vi "Load LVS EMA 2010b.vi"(10 "Data OUT in":T1={"Impulse Positions"=[], "Old Impulse positions for Undo"=[], "No. Imp"=0, "Parameter Time Series"=[], "Parameter Impuls Series"=[], "Experiment Parameters"={"Freq"=0.0, "Vel"=0, "Acc"=0, "Stimulus"=""}, "Autosort File"=refnum, "Data File"={"Data Channels"=[], "Sample Rate"=0, "Channel List"=[]}, "Experiment data path"=path "", "Image data path"=path "", "LVS data path"=path "", "Raw copy path"=path "", "filename"="", "desaccading parameters"={"Tolerance"=0, "Acc Range"=0.0, "Sample Rate"=0, "Impulse Plane 2"=enum."Other", "Impulse dir"=FALSE}, "Experiment Parameters 2"={"Subject"="", "Strain"="", "Rotation plane"="", "Experimenter"="", "Trial"=0.0, "Time"=0.0}, "Excel"={"Excel._Application"=refnum, "Use Excel"=FALSE, "Worksheet SINE"=refnum, "Row SINE"=0, "Worksheet TRANS"=refnum, "Row TRANS"=0}, "Session Config File"=refnum, "Autosort Parameter Set"=0, "EMA Version"="", "desacc "={"Threshold 1 [Acc]"=0.0, "Threshold 2 [% of TH1]"=0, "tolerance"=0, "Search WD "=0.0, " always use TH2"=FALSE, "Range"=0.0, "Max time"=0.0, "Min time"=0.0, "Velocity Threshold"=0}, "Cycle Nr for Saccades"={"POS"=0, "NEG"=0}, "Undo Counter"=0, "History Length"=0, "Redo Counter"=0, "Histpry Position"=0, "Raw Data File"={"Data Channels"=[], "Sample Rate"=0, "Channel List"=[]}, "calibration name"="No file selected"} {"Parameter Time Series"."time offset" format="%.3f"; "Parameter Time Series"."Gain" format="%.1f"; "Parameter Time Series"."Offset" format="%.1f"; "Parameter Time Series"."List 1" items=["Motor-Pos", "Motor-Vel", "Lx Position-in-Head", "Ly Position-in-Head", "Lz Position-in-Head", "Lx Velocity-in-Head", "Ly Velocity-in-Head", "Lz Velocity-in-Head", "Ll Velocity-in-Head", "Lr Velocity-in-Head", "Lx Accel-in-Head", "Ly Accel-in-Head", "Lz Accel-in-Head", "Rx Position-in-Head", "Ry Position-in-Head", "Rz Position-in-Head", "Rx Velocity-in-Head", "Ry Velocity-in-Head", "Rz Velocity-in-Head", "Rl Velocity-in-Head", "Rr Velocity-in-Head", "Rx Accel-in-Head", "Ry Accel-in-Head", "Rz Accel-in-Head", "Global Trigger", "", "", ""]; "Parameter Impuls Series"."Gain" format="%.1f"; "Parameter Impuls Series"."Offset" format="%.1f"}, 11 "Byte Stream File in":refnum<file>) -> (2 "Byte Stream File out":refnum<file>, 3 "Data OUT out":T1={"Impulse Positions"=[], "Old Impulse positions for Undo"=[], "No. Imp"=0, "Parameter Time Series"=[], "Parameter Impuls Series"=[], "Experiment Parameters"={"Freq"=0.0, "Vel"=0, "Acc"=0, "Stimulus"=""}, "Autosort File"=refnum, "Data File"={"Data Channels"=[], "Sample Rate"=0, "Channel List"=[]}, "Experiment data path"=path "", "Image data path"=path "", "LVS data path"=path "", "Raw copy path"=path "", "filename"="", "desaccading parameters"={"Tolerance"=0, "Acc Range"=0.0, "Sample Rate"=0, "Impulse Plane 2"=enum."Other", "Impulse dir"=FALSE}, "Experiment Parameters 2"={"Subject"="", "Strain"="", "Rotation plane"="", "Experimenter"="", "Trial"=0.0, "Time"=0.0}, "Excel"={"Excel._Application"=refnum, "Use Excel"=FALSE, "Worksheet SINE"=refnum, "Row SINE"=0, "Worksheet TRANS"=refnum, "Row TRANS"=0}, "Session Config File"=refnum, "Autosort Parameter Set"=0, "EMA Version"="", "desacc "={"Threshold 1 [Acc]"=0.0, "Threshold 2 [% of TH1]"=0, "tolerance"=0, "Search WD "=0.0, " always use TH2"=FALSE, "Range"=0.0, "Max time"=0.0, "Min time"=0.0, "Velocity Threshold"=0}, "Cycle Nr for Saccades"={"POS"=0, "NEG"=0}, "Undo Counter"=0, "History Length"=0, "Redo Counter"=0, "Histpry Position"=0, "Raw Data File"={"Data Channels"=[], "Sample Rate"=0, "Channel List"=[]}, "calibration name"="No file selected"} {"Parameter Time Series"."time offset" format="%.3f"; "Parameter Time Series"."Gain" format="%.1f"; "Parameter Time Series"."Offset" format="%.1f"; "Parameter Time Series"."List 1" items=["Motor-Pos", "Motor-Vel", "Lx Position-in-Head", "Ly Position-in-Head", "Lz Position-in-Head", "Lx Velocity-in-Head", "Ly Velocity-in-Head", "Lz Velocity-in-Head", "Ll Velocity-in-Head", "Lr Velocity-in-Head", "Lx Accel-in-Head", "Ly Accel-in-Head", "Lz Accel-in-Head", "Rx Position-in-Head", "Ry Position-in-Head", "Rz Position-in-Head", "Rx Velocity-in-Head", "Ry Velocity-in-Head", "Rz Velocity-in-Head", "Rl Velocity-in-Head", "Rr Velocity-in-Head", "Rx Accel-in-Head", "Ry Accel-in-Head", "Rz Accel-in-Head", "Global Trigger", "", "", ""]; "Parameter Impuls Series"."Gain" format="%.1f"; "Parameter Impuls Series"."Offset" format="%.1f"})   [LabVIEW 2014]
uses:
  type-defs/TD_Statemachine-Data.ctl
  type-defs/TD_Time Series.ctl
  type-defs/TD_Impulse Parameter.ctl
  core.lvlib
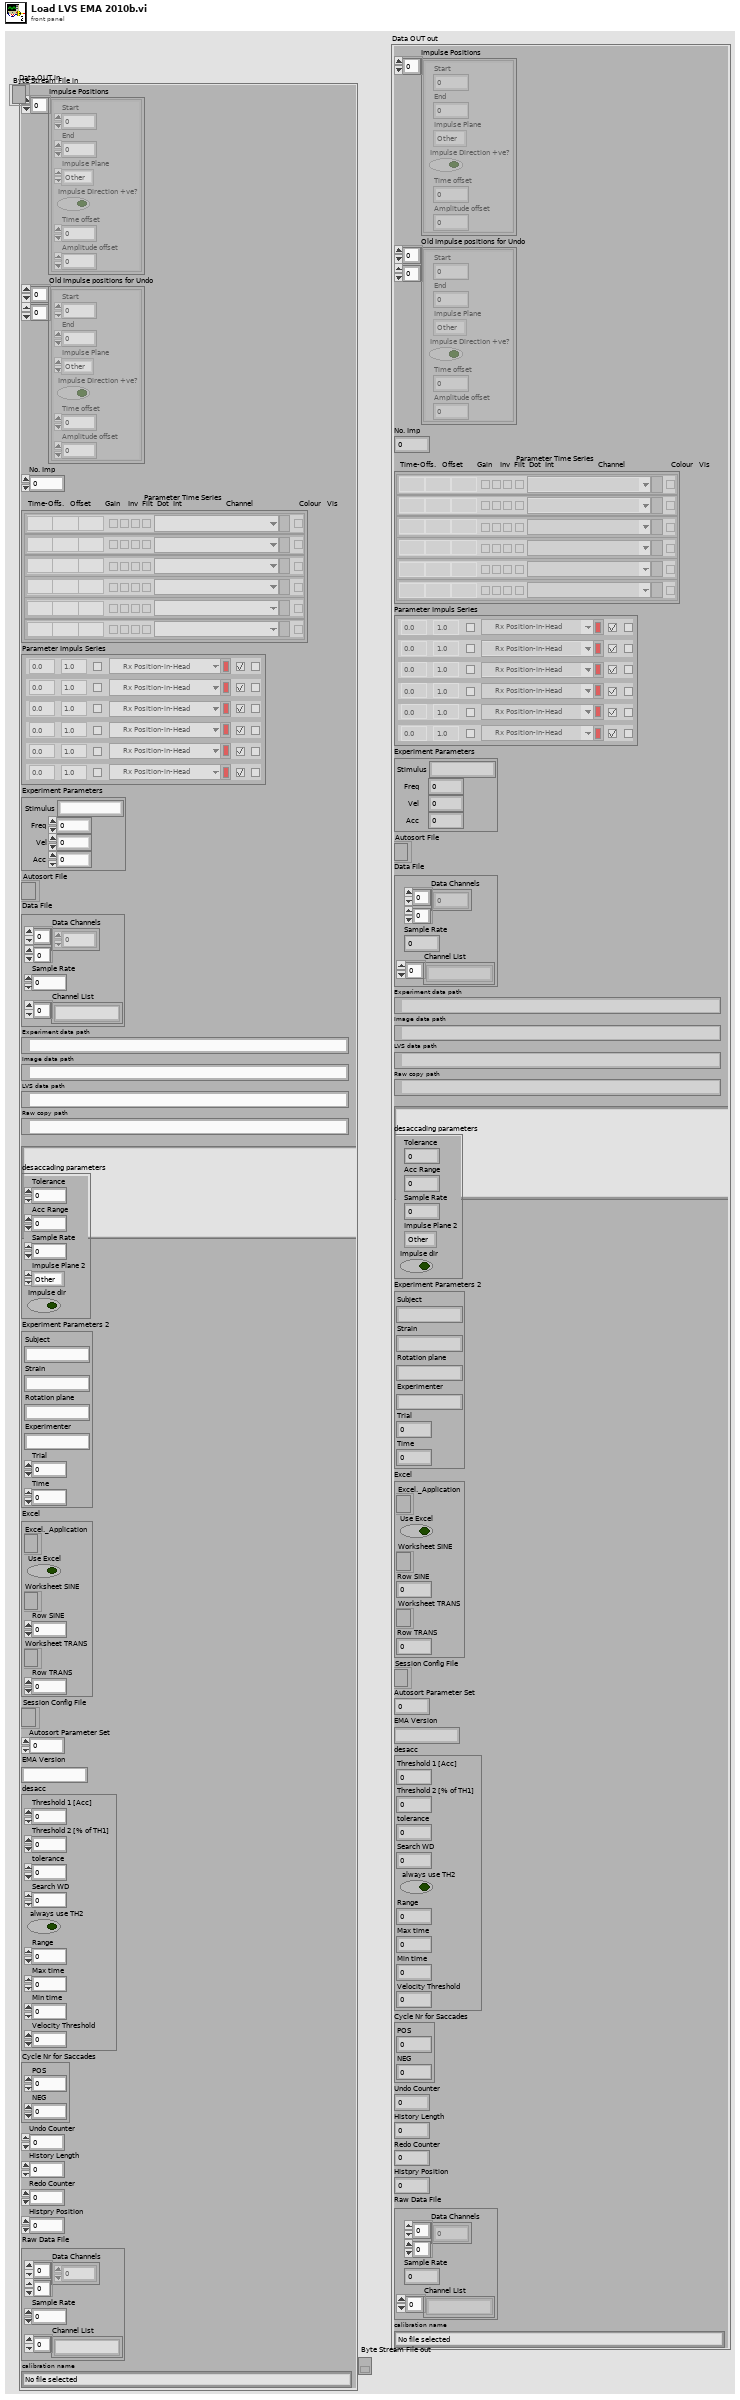
[diagram p1: front panel]
types:
  T1 = typedef "core.lvlib/TD_Statemachine-Data.ctl" = cluster{"Impulse Positions":cluster{"Start":i32, "End":i32, "Impulse Plane":enum16{"Other", "Yaw", "Pitch", "Roll", "LARP", "RALP"}, "Impulse Direction +ve?":bool, "Time offset":i32, "Amplitude offset":dbl}[], "Old Impulse positions for Undo":cluster{"Start":i32, "End":i32, "Impulse Plane":enum16{"Other", "Yaw", "Pitch", "Roll", "LARP", "RALP"}, "Impulse Direction +ve?":bool, "Time offset":i32, "Amplitude offset":dbl}[][], "No. Imp":i32, "Parameter Time Series":T2, "Parameter Impuls Series":T3, "Experiment Parameters":cluster{"Freq":dbl, "Vel":i32, "Acc":i32, "Stimulus":string}, "Autosort File":refnum<file>, "Data File":cluster{"Data Channels":dbl[][], "Sample Rate":i32, "Channel List":string[]}, "Experiment data path":path, "Image data path":path, "LVS data path":path, "Raw copy path":path, "filename":string, "desaccading parameters":cluster{"Tolerance":i32, "Acc Range":dbl, "Sample Rate":i32, "Impulse Plane 2":enum16{"Other", "Yaw", "Pitch", "Roll", "LARP", "RALP"}, "Impulse dir":bool}, "Experiment Parameters 2":cluster{"Subject":string, "Strain":string, "Rotation plane":string, "Experimenter":string, "Trial":dbl, "Time":dbl}, "Excel":cluster{"Excel._Application":refnum<k7>, "Use Excel":bool, "Worksheet SINE":refnum<k7>, "Row SINE":i32, "Worksheet TRANS":refnum<k7>, "Row TRANS":i32}, "Session Config File":refnum<file>, "Autosort Parameter Set":i32, "EMA Version":string, "desacc ":cluster{"Threshold 1 [Acc]":dbl, "Threshold 2 [% of TH1]":i32, "tolerance":i32, "Search WD ":dbl, " always use TH2":bool, "Range":dbl, "Max time":dbl, "Min time":dbl, "Velocity Threshold":i32}, "Cycle Nr for Saccades":cluster{"POS":i32, "NEG":i32}, "Undo Counter":i32, "History Length":i32, "Redo Counter":i32, "Histpry Position":i32, "Raw Data File":cluster{"Data Channels":dbl[][], "Sample Rate":i32, "Channel List":string[]}, "calibration name":string}
  T2 = typedef "core.lvlib/TD_Time Series.ctl" = cluster{"time offset":dbl, "Offset":dbl, "Gain":dbl, "inverse":bool, "filter data":bool, "dots":bool, "interpolate":bool, "List 1":u16, "Color Box":u32, "Boolean":bool}[]
  T3 = typedef "core.lvlib/TD_Impulse Parameter.ctl" = cluster{"Color":u32, "Visible":bool, "Channel":u16, "Invert":bool, "Desaccade":bool, "Offset":dbl, "Gain":dbl}[]
  T4 = cluster{"Data Channels":dbl[][], "Sample Rate":i32, "Channel List":string[]}
  T5 = cluster{"Data Output":cluster{"Data Channels":dbl[][], "Sample Rate":i32, "Channel List":string[]}, "Data OUT in":T1}
  T6 = cluster{"Start":i32, "End":i32, "Impulse Plane":enum16{"Other", "Yaw", "Pitch", "Roll", "LARP", "RALP"}, "Impulse Direction +ve?":bool, "Time offset":i32, "Amplitude offset":dbl}[]
  T7 = cluster{"Start":i32, "End":i32, "Impulse Plane":enum16{"Other", "Yaw", "Pitch", "Roll", "LARP", "RALP"}, "Impulse Direction +ve?":bool, "Time offset":i32, "Amplitude offset":dbl}[][]
  T8 = cluster{"Freq":dbl, "Vel":i32, "Acc":i32, "Stimulus":string}
  T9 = cluster{"Tolerance":i32, "Acc Range":dbl, "Sample Rate":i32, "Impulse Plane 2":enum16{"Other", "Yaw", "Pitch", "Roll", "LARP", "RALP"}, "Impulse dir":bool}
  T10 = cluster{"Subject":string, "Strain":string, "Rotation plane":string, "Experimenter":string, "Trial":dbl, "Time":dbl}
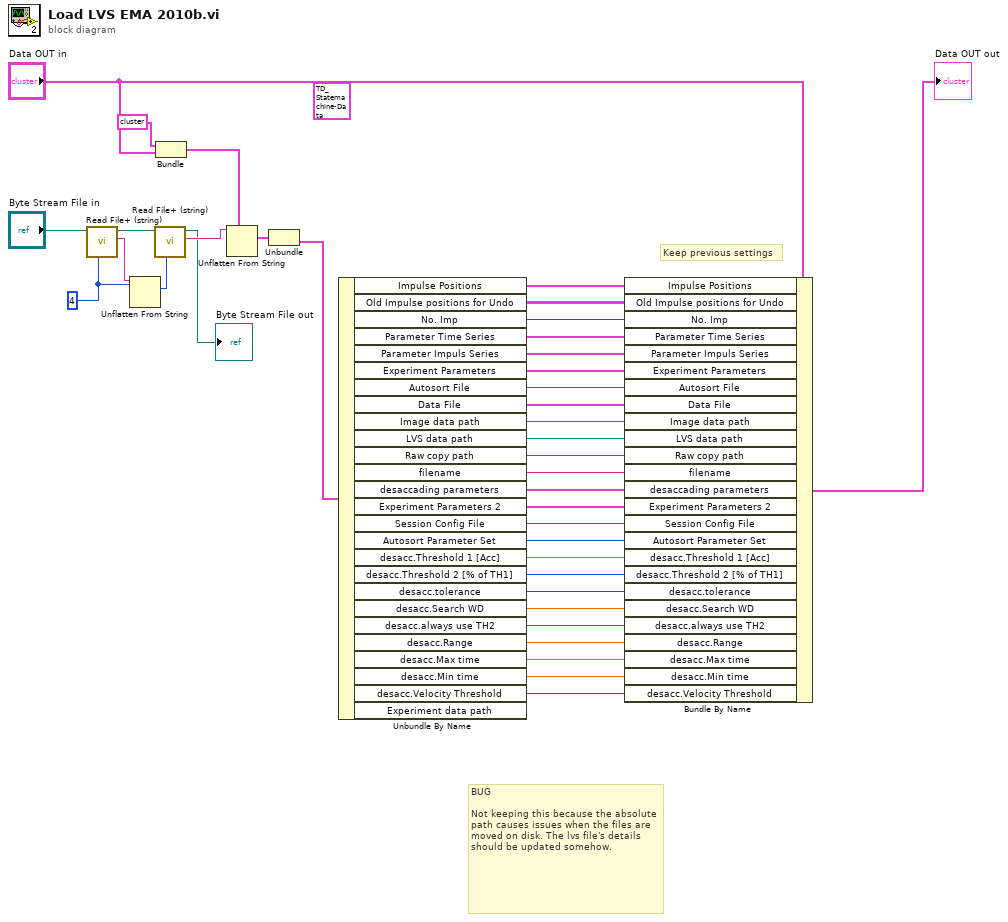
[diagram p0: block diagram]
diagram:
  (unwired) T1 {"Impulse Positions"=[{"Start"=4942, "End"=5034, "Impulse Plane"=enum."Yaw", "Impulse Direction +ve?"=TRUE, "Time offset"=0, "Amplitude offset"=0.0}, {"Start"=5524, "End"=5615, "Impulse Plane"=enum."Yaw", "Impulse Direction +ve?"=FALSE, "Time offset"=0, "Amplitude offset"=0.0}, {"Start"=6320, "End"=6414, "Impulse Plane"=enum."Yaw", "Impulse Direction +ve?"=FALSE, "Time offset"=0, "Amplitude offset"=0.0}, {"Start"=6789, "End"=6880, "Impulse Plane"=enum."Yaw", "Impulse Direction +ve?"=TRUE, "Time offset"=0, "Amplitude offset"=0.0}, {"Start"=7275, "End"=7365, "Impulse Plane"=enum."Yaw", "Impulse Direction +ve?"=FALSE, "Time offset"=0, "Amplitude offset"=0.0}, {"Start"=7765, "End"=7854, "Impulse Plane"=enum."Yaw", "Impulse Direction +ve?"=FALSE, "Time offset"=0, "Amplitude offset"=0.0}, {"Start"=8262, "End"=8354, "Impulse Plane"=enum."Yaw", "Impulse Direction +ve?"=TRUE, "Time offset"=0, "Amplitude offset"=0.0}, {"Start"=9102, "End"=9192, "Impulse Plane"=enum."Yaw", "Impulse Direction +ve?"=TRUE, "Time offset"=0, "Amplitude offset"=0.0}, {"Start"=9641, "End"=9736, "Impulse Plane"=enum."Yaw", "Impulse Direction +ve?"=FALSE, "Time offset"=0, "Amplitude offset"=0.0}, {"Start"=10150, "End"=10242, "Impulse Plane"=enum."Yaw", "Impulse Direction +ve?"=FALSE, "Time offset"=0, "Amplitude offset"=0.0}, {"Start"=10613, "End"=10703, "Impulse Plane"=enum."Yaw", "Impulse Direction +ve?"=TRUE, "Time offset"=0, "Amplitude offset"=0.0}, {"Start"=11147, "End"=11237, "Impulse Plane"=enum."Yaw", "Impulse Direction +ve?"=TRUE, "Time offset"=0, "Amplitude offset"=0.0}, {"Start"=11689, "End"=11781, "Impulse Plane"=enum."Yaw", "Impulse Direction +ve?"=TRUE, "Time offset"=0, "Amplitude offset"=0.0}, {"Start"=12321, "End"=12416, "Impulse Plane"=enum."Yaw", "Impulse Direction +ve?"=FALSE, "Time offset"=0, "Amplitude offset"=0.0}, {"Start"=12810, "End"=12901, "Impulse Plane"=enum."Yaw", "Impulse Direction +ve?"=FALSE, "Time offset"=0, "Amplitude offset"=0.0}, {"Start"=13306, "End"=13397, "Impulse Plane"=enum."Yaw", "Impulse Direction +ve?"=FALSE, "Time offset"=0, "Amplitude offset"=0.0}, {"Start"=13888, "End"=13980, "Impulse Plane"=enum."Yaw", "Impulse Direction +ve?"=TRUE, "Time offset"=0, "Amplitude offset"=0.0}, {"Start"=14402, "End"=14493, "Impulse Plane"=enum."Yaw", "Impulse Direction +ve?"=FALSE, "Time offset"=0, "Amplitude offset"=0.0}, {"Start"=14971, "End"=15063, "Impulse Plane"=enum."Yaw", "Impulse Direction +ve?"=FALSE, "Time offset"=0, "Amplitude offset"=0.0}, {"Start"=15459, "End"=15553, "Impulse Plane"=enum."Yaw", "Impulse Direction +ve?"=TRUE, "Time offset"=0, "Amplitude offset"=0.0}, {"Start"=16020, "End"=16112, "Impulse Plane"=enum."Yaw", "Impulse Direction +ve?"=FALSE, "Time offset"=0, "Amplitude offset"=0.0}, {"Start"=16530, "End"=16622, "Impulse Plane"=enum."Yaw", "Impulse Direction +ve?"=TRUE, "Time offset"=0, "Amplitude offset"=0.0}, {"Start"=17204, "End"=17295, "Impulse Plane"=enum."Yaw", "Impulse Direction +ve?"=TRUE, "Time offset"=0, "Amplitude offset"=0.0}, {"Start"=17830, "End"=17921, "Impulse Plane"=enum."Yaw", "Impulse Direction +ve?"=FALSE, "Time offset"=0, "Amplitude offset"=0.0}, {"Start"=19274, "End"=19361, "Impulse Plane"=enum."Yaw", "Impulse Direction +ve?"=FALSE, "Time offset"=0, "Amplitude offset"=0.0}, {"Start"=19884, "End"=19973, "Impulse Plane"=enum."Yaw", "Impulse Direction +ve?"=FALSE, "Time offset"=0, "Amplitude offset"=0.0}, {"Start"=20423, "End"=20518, "Impulse Plane"=enum."Yaw", "Impulse Direction +ve?"=TRUE, "Time offset"=0, "Amplitude offset"=0.0}, {"Start"=21003, "End"=21091, "Impulse Plane"=enum."Yaw", "Impulse Direction +ve?"=FALSE, "Time offset"=0, "Amplitude offset"=0.0}, {"Start"=21526, "End"=21619, "Impulse Plane"=enum."Yaw", "Impulse Direction +ve?"=FALSE, "Time offset"=0, "Amplitude offset"=0.0}, {"Start"=22032, "End"=22124, "Impulse Plane"=enum."Yaw", "Impulse Direction +ve?"=TRUE, "Time offset"=0, "Amplitude offset"=0.0}, {"Start"=22661, "End"=22752, "Impulse Plane"=enum."Yaw", "Impulse Direction +ve?"=FALSE, "Time offset"=0, "Amplitude offset"=0.0}, {"Start"=23810, "End"=23900, "Impulse Plane"=enum."Yaw", "Impulse Direction +ve?"=TRUE, "Time offset"=0, "Amplitude offset"=0.0}], "Old Impulse positions for Undo"=[], "No. Imp"=18, "Parameter Time Series"=[{"time offset"=0.0, "Offset"=0.0, "Gain"=1.0, "inverse"=FALSE, "filter data"=FALSE, "dots"=FALSE, "interpolate"=FALSE, "List 1"=1, "Color Box"=65295, "Boolean"=TRUE}, {"time offset"=0.0, "Offset"=0.0, "Gain"=1.0, "inverse"=FALSE, "filter data"=FALSE, "dots"=FALSE, "interpolate"=FALSE, "List 1"=13, "Color Box"=16777224, "Boolean"=TRUE}, {"time offset"=0.0, "Offset"=0.0, "Gain"=1.0, "inverse"=FALSE, "filter data"=FALSE, "dots"=FALSE, "interpolate"=FALSE, "List 1"=6, "Color Box"=6618880, "Boolean"=FALSE}, {"time offset"=0.0, "Offset"=0.0, "Gain"=1.0, "inverse"=FALSE, "filter data"=FALSE, "dots"=FALSE, "interpolate"=FALSE, "List 1"=14, "Color Box"=16777224, "Boolean"=FALSE}, {"time offset"=0.0, "Offset"=0.0, "Gain"=1.0, "inverse"=FALSE, "filter data"=FALSE, "dots"=FALSE, "interpolate"=FALSE, "List 1"=7, "Color Box"=6618880, "Boolean"=FALSE}, {"time offset"=0.0, "Offset"=0.0, "Gain"=1.0, "inverse"=FALSE, "filter data"=FALSE, "dots"=FALSE, "interpolate"=FALSE, "List 1"=15, "Color Box"=16777224, "Boolean"=FALSE}], "Parameter Impuls Series"=[{"Color"=4652800, "Visible"=TRUE, "Channel"=1, "Invert"=FALSE, "Desaccade"=FALSE, "Offset"=0.0, "Gain"=1.0}, {"Color"=16777224, "Visible"=TRUE, "Channel"=13, "Invert"=FALSE, "Desaccade"=FALSE, "Offset"=0.0, "Gain"=1.0}], "Experiment Parameters"={"Freq"=0.0, "Vel"=0, "Acc"=0, "Stimulus"="HIT-Lateral"}, "Autosort File"=refnum, "Data File"={"Data Channels"=array24x4503[108072 elements], "Sample Rate"=221, "Channel List"=["-", "Hz Velocity-in-Head", "-", "Hy Velocity-in-Head", "-", "Hx Velocity-in-Head", "Hl Velocity-in-Head", "Hr Velocity-in-Head", "Lx Position-in-Head", "Ly Position-in-Head", "Lz Position-in-Head", "Lx Velocity-in-Head", "Ly Velocity-in-Head", "Lz Velocity-in-Head", "Ll Velocity-in-Head", "Lr Velocity-in-Head", "-", "-", "-", "-", "-", "-", "-", "-"]}, "Experiment data path"=path "C:/Users/w.figtree/Desktop/Subject 10/Day 4", "Image data path"=path "", "LVS data path"=path "", "Raw copy path"=path "", "filename"="p00001s003e016c001t003.mat", "desaccading parameters"={"Tolerance"=0, "Acc Range"=0.0, "Sample Rate"=221, "Impulse Plane 2"=enum."Yaw", "Impulse dir"=FALSE}, "Experiment Parameters 2"={"Subject"="SE Trial Short Term", "Strain"="", "Rotation plane"="", "Experimenter"=" ", "Trial"=0.0, "Time"=0.0}, "Excel"={"Excel._Application"=refnum, "Use Excel"=TRUE, "Worksheet SINE"=refnum, "Row SINE"=0, "Worksheet TRANS"=refnum, "Row TRANS"=0}, "Session Config File"=refnum, "Autosort Parameter Set"=10, "EMA Version"="EMA 2011b", "desacc "={"Threshold 1 [Acc]"=0.0, "Threshold 2 [% of TH1]"=0, "tolerance"=0, "Search WD "=0.0, " always use TH2"=FALSE, "Range"=0.0, "Max time"=0.0, "Min time"=0.0, "Velocity Threshold"=0}, "Cycle Nr for Saccades"={"POS"=0, "NEG"=0}, "Undo Counter"=0, "History Length"=0, "Redo Counter"=0, "Histpry Position"=-1, "Raw Data File"={"Data Channels"=[], "Sample Rate"=0, "Channel List"=[]}, "calibration name"="p00001s003_calib.mat"} ("Data OUT in")
  w5 = 4 ("count")
  # "BUG\n\nNot keeping this because the absolute path causes issues when the files are moved on disk. The lvs file's details should be updated somehow."
  # "Keep previous settings"
  n1 = call <vilib>:"Read File+ (string).vi"("count"=w5, "refnum"="Byte Stream File in") -> ("string"=w4:string, "dup refnum"=w3:refnum<file>)  [unwired: 5 in, 3 out]
  n2 = Unflatten From String(type=w5, binary string=w4) -> (value=w6:i32)  [unwired: 3 in, 2 out]
  n3 = call <vilib>:"Read File+ (string).vi"("count"=w6, "refnum"=w3) -> ("string"=w2:string, "dup refnum"=→"Byte Stream File out":refnum<file>)  [unwired: 5 in, 3 out]
  n4 = Bundle("Data Output"=T4 {"Data Channels"=array28x10017[280476 elements], "Sample Rate"=200, "Channel List"=["Motor-Pos", "Motor-Vel", "Lx Position-in-Head", "Ly Position-in-Head", "Lz Position-in-Head", "Lx Velocity-in-Head", "Ly Velocity-in-Head", "Lz Velocity-in-Head", "Ll Velocity-in-Head", "Lr Velocity-in-Head", "Lx Accel-in-Head", "Ly Accel-in-Head", "Lz Accel-in-Head", "Rx Position-in-Head", "Ry Position-in-Head", "Rz Position-in-Head", "Rx Velocity-in-Head", "Ry Velocity-in-Head", "Rz Velocity-in-Head", "Rl Velocity-in-Head", "Rr Velocity-in-Head", "Rx Accel-in-Head", "Ry Accel-in-Head", "Rz Accel-in-Head", "Global Trigger", "\tNA", "\tNA", "\tNA"]}, "Data OUT in"="Data OUT in") -> (w7:T5)  [unwired: 1 in]
  n5 = Unflatten From String(type=w7, binary string=w2) -> (value=w8:T5)  [unwired: 3 in, 2 out]
  n6 = Unbundle(w8) -> ("Data OUT in"=w11:T1)  [unwired: 1 out]
  n7 = Unbundle By Name(w11) -> ("Impulse Positions"=w12:T6, "Old Impulse positions for Undo"=w13:T7, "No. Imp"=w14:i32, "Parameter Time Series"=w15:T2, "Parameter Impuls Series"=w16:T3, "Experiment Parameters"=w17:T8, "Autosort File"=w18:refnum<file>, "Data File"=w19:T4, "Image data path"=w20:path, "LVS data path"=w21:path, "Raw copy path"=w22:path, "filename"=w23:string, "desaccading parameters"=w24:T9, "Experiment Parameters 2"=w25:T10, "Session Config File"=w26:refnum<file>, "Autosort Parameter Set"=w27:i32, "desacc.Threshold 1 [Acc]"=w28:dbl, "desacc.Threshold 2 [% of TH1]"=w29:i32, "desacc.tolerance"=w30:i32, "desacc.Search WD"=w31:dbl, "desacc.always use TH2"=w32:bool, "desacc.Range"=w33:dbl, "desacc.Max time"=w34:dbl, "desacc.Min time"=w35:dbl, "desacc.Velocity Threshold"=w37:i32)  [unwired: 1 out]
  n8 = Bundle By Name(cluster="Data OUT in", "Impulse Positions"=w12, "Old Impulse positions for Undo"=w13, "No. Imp"=w14, "Parameter Time Series"=w15, "Parameter Impuls Series"=w16, "Experiment Parameters"=w17, "Autosort File"=w18, "Data File"=w19, "Image data path"=w20, "LVS data path"=w21, "Raw copy path"=w22, "filename"=w23, "desaccading parameters"=w24, "Experiment Parameters 2"=w25, "Session Config File"=w26, "Autosort Parameter Set"=w27, "desacc.Threshold 1 [Acc]"=w28, "desacc.Threshold 2 [% of TH1]"=w29, "desacc.tolerance"=w30, "desacc.Search WD"=w31, "desacc.always use TH2"=w32, "desacc.Range"=w33, "desacc.Max time"=w34, "desacc.Min time"=w35, "desacc.Velocity Threshold"=w37) -> (→"Data OUT out":T1)
